vi "Launch Service Monitor.vi"(0 "Room Service Monitor Model in":refnum<class "Room Service Monitor Model.lvclass">, 5 "Service ID":string, 7 "Staff Name":string, 9 "Description":string, 11 "error in (no error)":errorcluster) -> (4 "Room Service Monitor Model out":refnum<class "Room Service Monitor Model.lvclass">, 15 "error out":errorcluster)   [LabVIEW 2023, in "Room Service Monitor Model.lvlib" / "Room Service Monitor Model.lvclass"]
uses:
  Room Service Monitor Model.lvclass
  Room Service Monitor Model.lvclass/Room Service Monitor Model.ctl
  <vilib>/ActorFramework/Actor/Actor.lvclass
  Room Service Monitor UI/Room Service Monitor UI/Room Service Monitor UI.lvclass
  C:/Users/bhaghyaraj/Trainings/NI Actor Framework/SDLC/UI Base/UI Base/UI Base.lvclass
  C:/Program Files/National Instruments/LabVIEW 2023/vi.lib/ActorFramework/Actor/Actor.lvclass
  C:/Users/bhaghyaraj/Trainings/NI Actor Framework/SDLC/Room Service Monitor UI/Room Service Monitor UI/Room Service Monitor UI.lvclass
  C:/Users/bhaghyaraj/Trainings/NI Actor Framework/SDLC/Model Base/Model Base/Model Base.lvclass
  C:/Users/bhaghyaraj/Trainings/NI Actor Framework/SDLC/Interfaces/Model Base/Incoming Model Base Interface.lvclass
  C:/Users/bhaghyaraj/Trainings/NI Actor Framework/SDLC/Room Service Monitor Model/Room Service Monitor Model/Room Service Monitor Model.lvclass
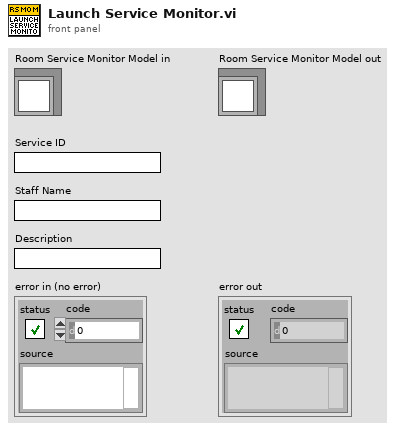
[diagram p1: front panel]
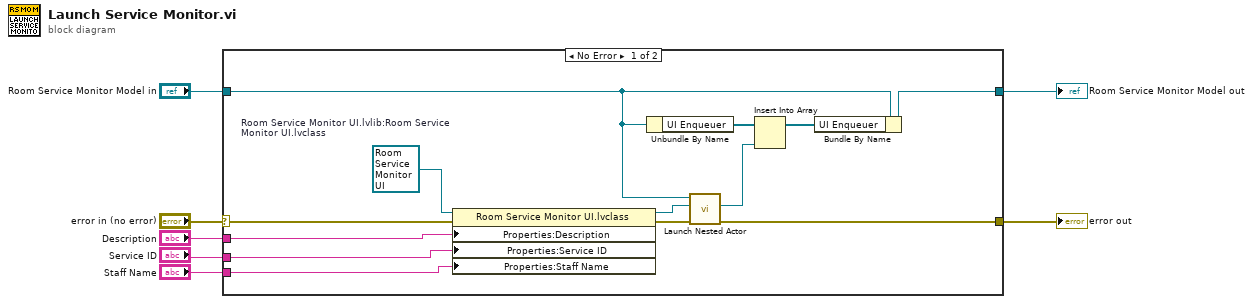
[diagram p0: block diagram]
diagram:
  n1 = case shown="No Error" "error in (no error)" {
    selector: "error in (no error)" -> [w20 w22]
    tunnel: [w19 w22] -> w6
    tunnel: [w14 w21] -> w4
    tunnel: "Room Service Monitor Model in" -> [w18 w21]
    tunnel: "Description" -> [w10 _]
    tunnel: "Service ID" -> [w9 _]
    tunnel: "Staff Name" -> [w8 _]
    frame No Error {
      w16 = refnum<class "Room Service Monitor UI.lvclass"> refnum  # Room Service Monitor UI.lvlib:Room Service Monitor UI.lvclass
      n2 = property class="Room Service Monitor UI.lvclass"(reference=w16, error in=w20, "Properties:Description"=w10, "Properties:Service ID"=w9, "Properties:Staff Name"=w8) -> (reference out=w15:refnum<class "Room Service Monitor UI.lvclass">, error out=w17:errorcluster)
      n3 = Unbundle By Name(w18) -> ("UI Enqueuer"=w13:refnum<class "Message Enqueuer.lvclass">[])
      n4 = call <vilib>:"Launch Nested Actor.vi"("error in (no error)"=w17, "Nested Actor"=w15, "Caller Actor in"=w18) -> ("error out"=w19:errorcluster, "Nested Actor's Enqueuer"=w11:refnum<class "Message Enqueuer.lvclass">)  [unwired: 6 in, 1 out]
      n5 = Insert Into Array(array=w13, new element=w11) -> (w12:refnum<class "Message Enqueuer.lvclass">[])  [unwired: 1 in]
      n6 = Bundle By Name(cluster=w18, "UI Enqueuer"=w12) -> (w14:refnum<class "Room Service Monitor Model.lvclass">)
    }
    frame Error {
    }
  }
  "error out" <- w6
  "Room Service Monitor Model out" <- w4
